vi "Equal.vi"() -> ()   [LabVIEW 2017, in "Assertions.Tests.lvlib" / "Assert Less Than.lvlib"]
uses:
  Assert Less Than.lvlib
  ca741bb9-a7b7-41c9-8e97-600369c8edc7.vi
  src/Transparent Assertions/Constraints/Is Less Than/Create.vi
  src/Transparent Assertions/Constraints/Is Less Than/Is Less Than.lvclass
  src/Transparent Assertions/Assertions/Assertions.lvlib
panel:
  out "error out":errorcluster
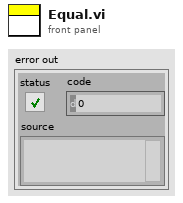
[diagram p1: front panel]
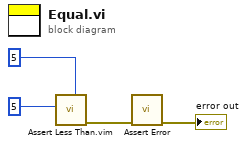
[diagram p0: block diagram]
diagram:
  n1 = call "Assert Less Than.vim"("Expected"=5, "Actual"=5) -> ("error out"=w2:errorcluster)  [unwired: 9 in]
  n2 = call "Assert Error.vi"("error in (no error)"=w2) -> ("error out"=→"error out":errorcluster)  [unwired: 10 in]
